vi "AlphaBetaToABC_src.vi"(0 "alpha":sgl format="%#_32g", 5 "beta":sgl format="%#_32g") -> (4 "A":sgl format="%#_32g", 6 "B":sgl, 8 "C":sgl)   [LabVIEW 2015]
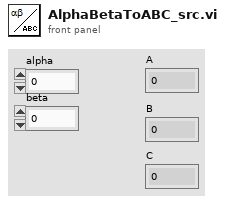
[diagram p1: front panel]
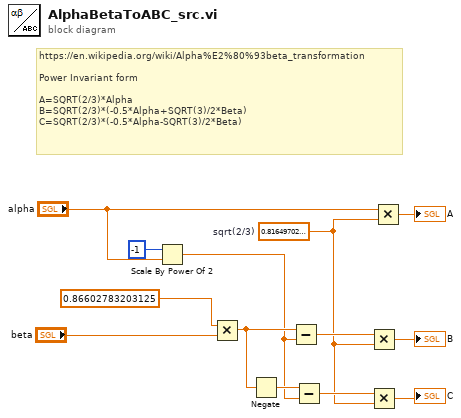
[diagram p0: block diagram]
diagram:
  w1 = sgl 0.816497  # sqrt(2/3)
  # "https://en.wikipedia.org/wiki/Alpha%E2%80%93beta_transformation\n\nPower Invariant form\n\nA=SQRT(2/3)*Alpha\nB=SQRT(2/3)*(-0.5*Alpha+SQRT(3)/2*Beta)\nC=SQRT(2/3)*(-0.5*Alpha-SQRT(3)/2*Beta)"
  n1 = Scale By Power Of 2(n=i16 -1, x="alpha") -> (x*2^n=w8:sgl)
  n2 = Multiply(x=sgl 0.86602783 ("beta"), y="beta") -> (x*y=w10:sgl)
  n3 = Negate(x=w10) -> (-x=w9:sgl)
  n4 = Subtract(x=w10, y=w8) -> (x-y=w4:sgl)
  n5 = Subtract(x=w9, y=w8) -> (x-y=w2:sgl)
  n6 = Multiply(x=w4, y=w1) -> (x*y=→"B":sgl)
  n7 = Multiply(x=w2, y=w1) -> (x*y=→"C":sgl)
  n8 = Multiply(x="alpha", y=w1) -> (x*y=→"A":sgl)
